vi "Data_Record_Example.vi"() -> ()   [LabVIEW 2020]
uses:
  resources/gclib32/gclib32.lvlib
panel:
  out "RPA":i32
  out "TPA":i32
  out "TIME":u16
  out "TTA":dbl
  in  "IP Address":string="192.168.1.77 --subscribe DR "
  out "error out":errorcluster
  in  "stop":bool
  # "This example is built for the DMC-4000. If you have a different controller, check your controller's User Manual to ensure that the Data Record mapping is correct before running this program."
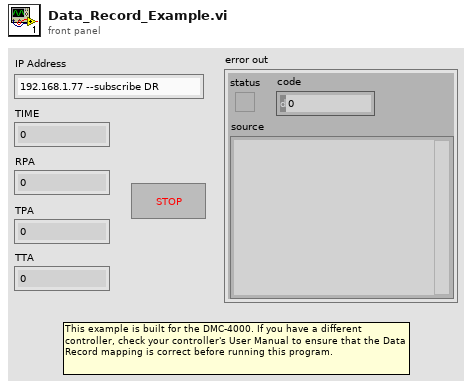
[diagram p1: front panel]
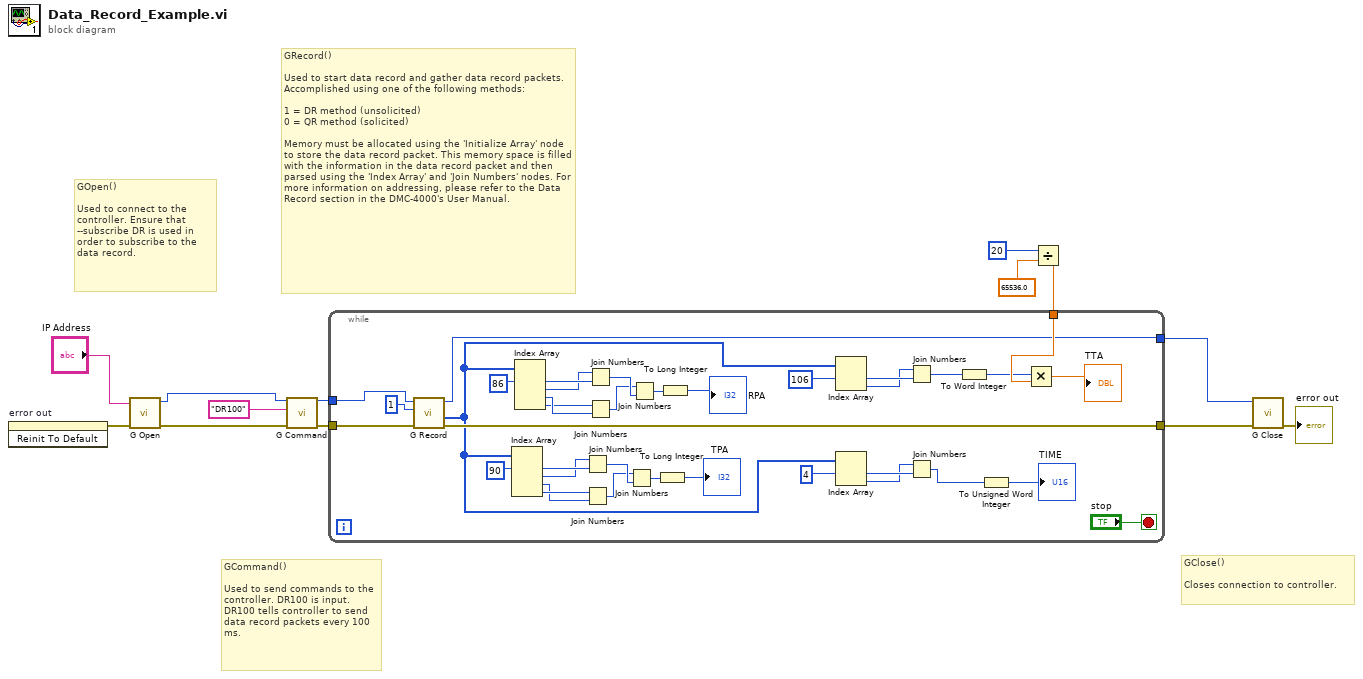
[diagram p0: block diagram]
diagram:
  # "GRecord()\n\nUsed to start data record and gather data record packets. Accomplished using one of the following methods:\n\n1 = DR method (unsolicited)\n0 = QR method (solicited)\n\nMemory must be allocated using the 'Initialize Array' node to store the data record packet. This memory space is filled with the information in the data record packet and then parsed using the 'Index Array' and 'Join Numbers' nodes. For more information on addressing, please refer to the Data Record section in the DMC-4000's User Manual."
  # "GClose()\n\nCloses connection to controller."
  # "GCommand()\n\nUsed to send commands to the controller. DR100 is input. DR100 tells controller to send data record packets every 100 ms."
  # "GOpen()\n\nUsed to connect to the controller. Ensure that \n--subscribe DR is used in order to subscribe to the data record."
  n1 = invoke on="error out" class="Clust (strict)" method="Reinit To Default"() -> (error out=w9:errorcluster)  [unwired: 3 in, 2 out]
  n2 = call "G Open.vi"("error in (no error)"=w9, "address"="IP Address") -> ("error out"=w5:errorcluster, "g out"=w7:u32)  [unwired: 7 in]
  n3 = call "G Command.vi"("g"=w7, "command"="DR100", "error in (no error)"=w5) -> ("g out"=w3:u32, "error out"=w4:errorcluster)  [unwired: 10 in, 1 out]
  n4 = Divide(x=20, y=65536.0) -> (x/y=w10:dbl)
  n5 = while {
    tunnel: [w16] -> w1
    tunnel: w3 -> [w19]
    tunnel: w4 -> [w18]
    tunnel: [w14] -> w2
    tunnel: w10 -> [w22]
    stop <- "stop" stop-if-true
    n6 = call "G Record.vi"("error in (no error)"=w18, "method"=1, "g"=w19) -> ("error out"=w16:errorcluster, "record out"=w15:u8[], "g out"=w14:u32)  [unwired: 6 in]
    n7 = Index Array "Index Array"(array=w15, index #1=90 ("index")) -> (element #1=w42:u8, element #2=w41:u8, element #3=w36:u8, element #4=w39:u8)  [unwired: 3 in]
    n8 = Index Array "Index Array"(array=w15, index #1=86 ("index")) -> (element #1=w49:u8, element #2=w48:u8, element #3=w46:u8, element #4=w45:u8)  [unwired: 3 in]
    n9 = Join Numbers(hi=w41, lo=w42) -> ((hi.lo)=w33:u16)
    n10 = Join Numbers(hi=w39, lo=w36) -> ((hi.lo)=w32:u16)
    n11 = Join Numbers(hi=w48, lo=w49) -> ((hi.lo)=w35:u16)
    n12 = Join Numbers(hi=w45, lo=w46) -> ((hi.lo)=w34:u16)
    n13 = Join Numbers(hi=w32, lo=w33) -> ((hi.lo)=w38:u32)
    n14 = Join Numbers(hi=w34, lo=w35) -> ((hi.lo)=w44:u32)
    n15 = To Long Integer(number=w38) -> (32bit integer=→"TPA":i32)
    n16 = To Long Integer(number=w44) -> (32bit integer=→"RPA":i32)
    n17 = Index Array "Index Array"(array=w15, index #1=106 ("index")) -> (element #1=w31:u8, element #2=w30:u8)  [unwired: 1 in]
    n18 = Index Array "Index Array"(array=w15, index #1=4 ("index")) -> (element #1=w28:u8, element #2=w27:u8)  [unwired: 1 in]
    n19 = Join Numbers(hi=w30, lo=w31) -> ((hi.lo)=w23:u16)
    n20 = Join Numbers(hi=w27, lo=w28) -> ((hi.lo)=w25:u16)
    n21 = To Word Integer(number=w23) -> (16bit integer=w21:i16)
    n22 = To Unsigned Word Integer(number=w25) -> (unsigned 16bit integer=→"TIME":u16)
    n23 = Multiply(x=w21, y=w22) -> (x*y=→"TTA":dbl)
  }
  n24 = call "G Close.vi"("error in (no error)"=w1, "g"=w2) -> ("error out"=→"error out":errorcluster)  [unwired: 9 in]
